vi "LiftControlLoop.vi"() -> ()   [LabVIEW 2014, in "LiftLib.lvlib"]
uses:
  LiftLib.lvlib
  LiftRefs.ctl
  <vilib>/Rock Robotics/WPI/Solenoid/WPI_SolenoidValue.ctl
  <vilib>/addons/control/pid/pid.llb/PID (DBL).vi
  <vilib>/Rock Robotics/Network Tables/SD Write Number.vi
  <vilib>/Rock Robotics/Network Tables/SD Read Boolean.vi
  <vilib>/Rock Robotics/Network Tables/SD Write Boolean.vi
  <vilib>/addons/control/pid/NI_PID_pid.lvlib
  IntakeLib/IntakeLib.lvlib
panel:
  out "LiftRateLast":dbl format="%#_13g"
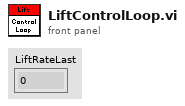
[diagram p1: front panel]
types:
  T1 = typedef "LiftLib.lvlib/LiftRefs.ctl" = enum16{"LiftCim1", "LiftCim2", "LiftEncoder", "LiftLimitSwitch1", "LiftLimitSwitch2"}
  T2 = typedef "WPI_MotorControlDeviceRef.ctl" = cluster{"DeviceStatus":errorcluster, "Type":T3, "PWM":cluster{"Controller":T4, "PWM Channel":T5, "DeadBand":T6}, "CAN":cluster{"Device Number":u8, "Control Mode":T7, "Semaphore":T8, "Max Vout":dbl, "TalonSRX Control Mode":T9}, "Invert":bool, "TransformRef":T10, "InvTransformRef":T10}
  T3 = typedef "WPI_MotorControlType.ctl" = enum16{"PWM", "CAN", "CANTalonSRX"}
  T4 = typedef "FPGA_TypedefDigitalModule.ctl" = enum16{"Controller 1"}
  T5 = typedef "FPGA_DIOPWMChannel.ctl" = enum8{"PWM 0", "PWM 1", "PWM 2", "PWM 3", "PWM 4", "PWM 5", "PWM 6", "PWM 7", "PWM 8", "PWM 9", "PWM MXP 0", "PWM MXP 1", "PWM MXP 2", "PWM MXP 3", "PWM MXP 4", "PWM MXP 5", "PWM MXP 6", "PWM MXP 7", "PWM MXP 8", "PWM MXP 9", "Invalid"}
  T6 = typedef "WPI_PWMDeadband.ctl" = cluster{"Name":string, "maxPositivePwm":i32, "minPositivePwm":i32, "centerPwm":i32, "maxNegativePwm":i32, "minNegativePwm":i32, "angularRange":u16}
  T7 = typedef "WPI_CANJaguar_ControlMode.ctl" = enum8{"Percent VBus", "Current", "Speed", "Position", "Voltage"}
  T8 = typedef "Semaphore RefNum" = refnum<k1>
  T9 = typedef "WPI_CANTalonSRX_APIControlMode.ctl" = enum8{"Percent VBus", "Speed", "Position", "Slave", "Unchanged / Invalid"}
  T10 = typedef "WPI_PWMTransform_ConPane.ctl" = refnum<vi>
  T11 = typedef "WPI_EncoderDevRef.ctl" = cluster{"DevStatus":errorcluster, "EncoderIndex":T12, "CounterIndex":T13, "DistancePerCount":dbl, "Decoding Type":T14}
  T12 = typedef "FPGA_EncoderIdx.ctl" = enum8{"Enc 0", "Enc 1", "Enc 2", "Enc 3", "Enc 4", "Enc 5", "Enc 6", "Enc 7", "Invalid"}
  T13 = typedef "FPGA_CounterCtrSystemIndex.ctl" = enum8{"Ctr 0", "Ctr 1", "Ctr 2", "Ctr 3", "Ctr 4", "Ctr 5", "Ctr 6", "Ctr 7", "Invalid"}
  T14 = typedef "WPI_EncoderType.ctl" = enum16{"1x", "2x", "4x"}
  T15 = typedef "WPI_DigitalInputDevRef.ctl" = cluster{"DevStatus":errorcluster, "DIO Channel":T16, "Controller":T4}
  T16 = typedef "FPGA_DIOChannel.ctl" = enum8{"DIO 0", "DIO 1", "DIO 2", "DIO 3", "DIO 4", "DIO 5", "DIO 6", "DIO 7", "DIO 8", "DIO 9", "DIO MXP 0", "DIO MXP 1", "DIO MXP 2", "DIO MXP 3", "DIO MXP 4", "DIO MXP 5", "DIO MXP 6", "DIO MXP 7", "DIO MXP 8", "DIO MXP 9", "DIO MXP 10", "DIO MXP 11", "DIO MXP 12", "DIO MXP 13", "DIO MXP 14", "DIO MXP 15", "Invalid"}
  T17 = typedef "WPI_SolenoidValue.ctl" = enum16{"Off", "On", "Forward", "Reverse"}
  T18 = cluster{"proportional gain (Kc)":dbl, "integral time (Ti, min)":dbl, "derivative time (Td, min)":dbl}
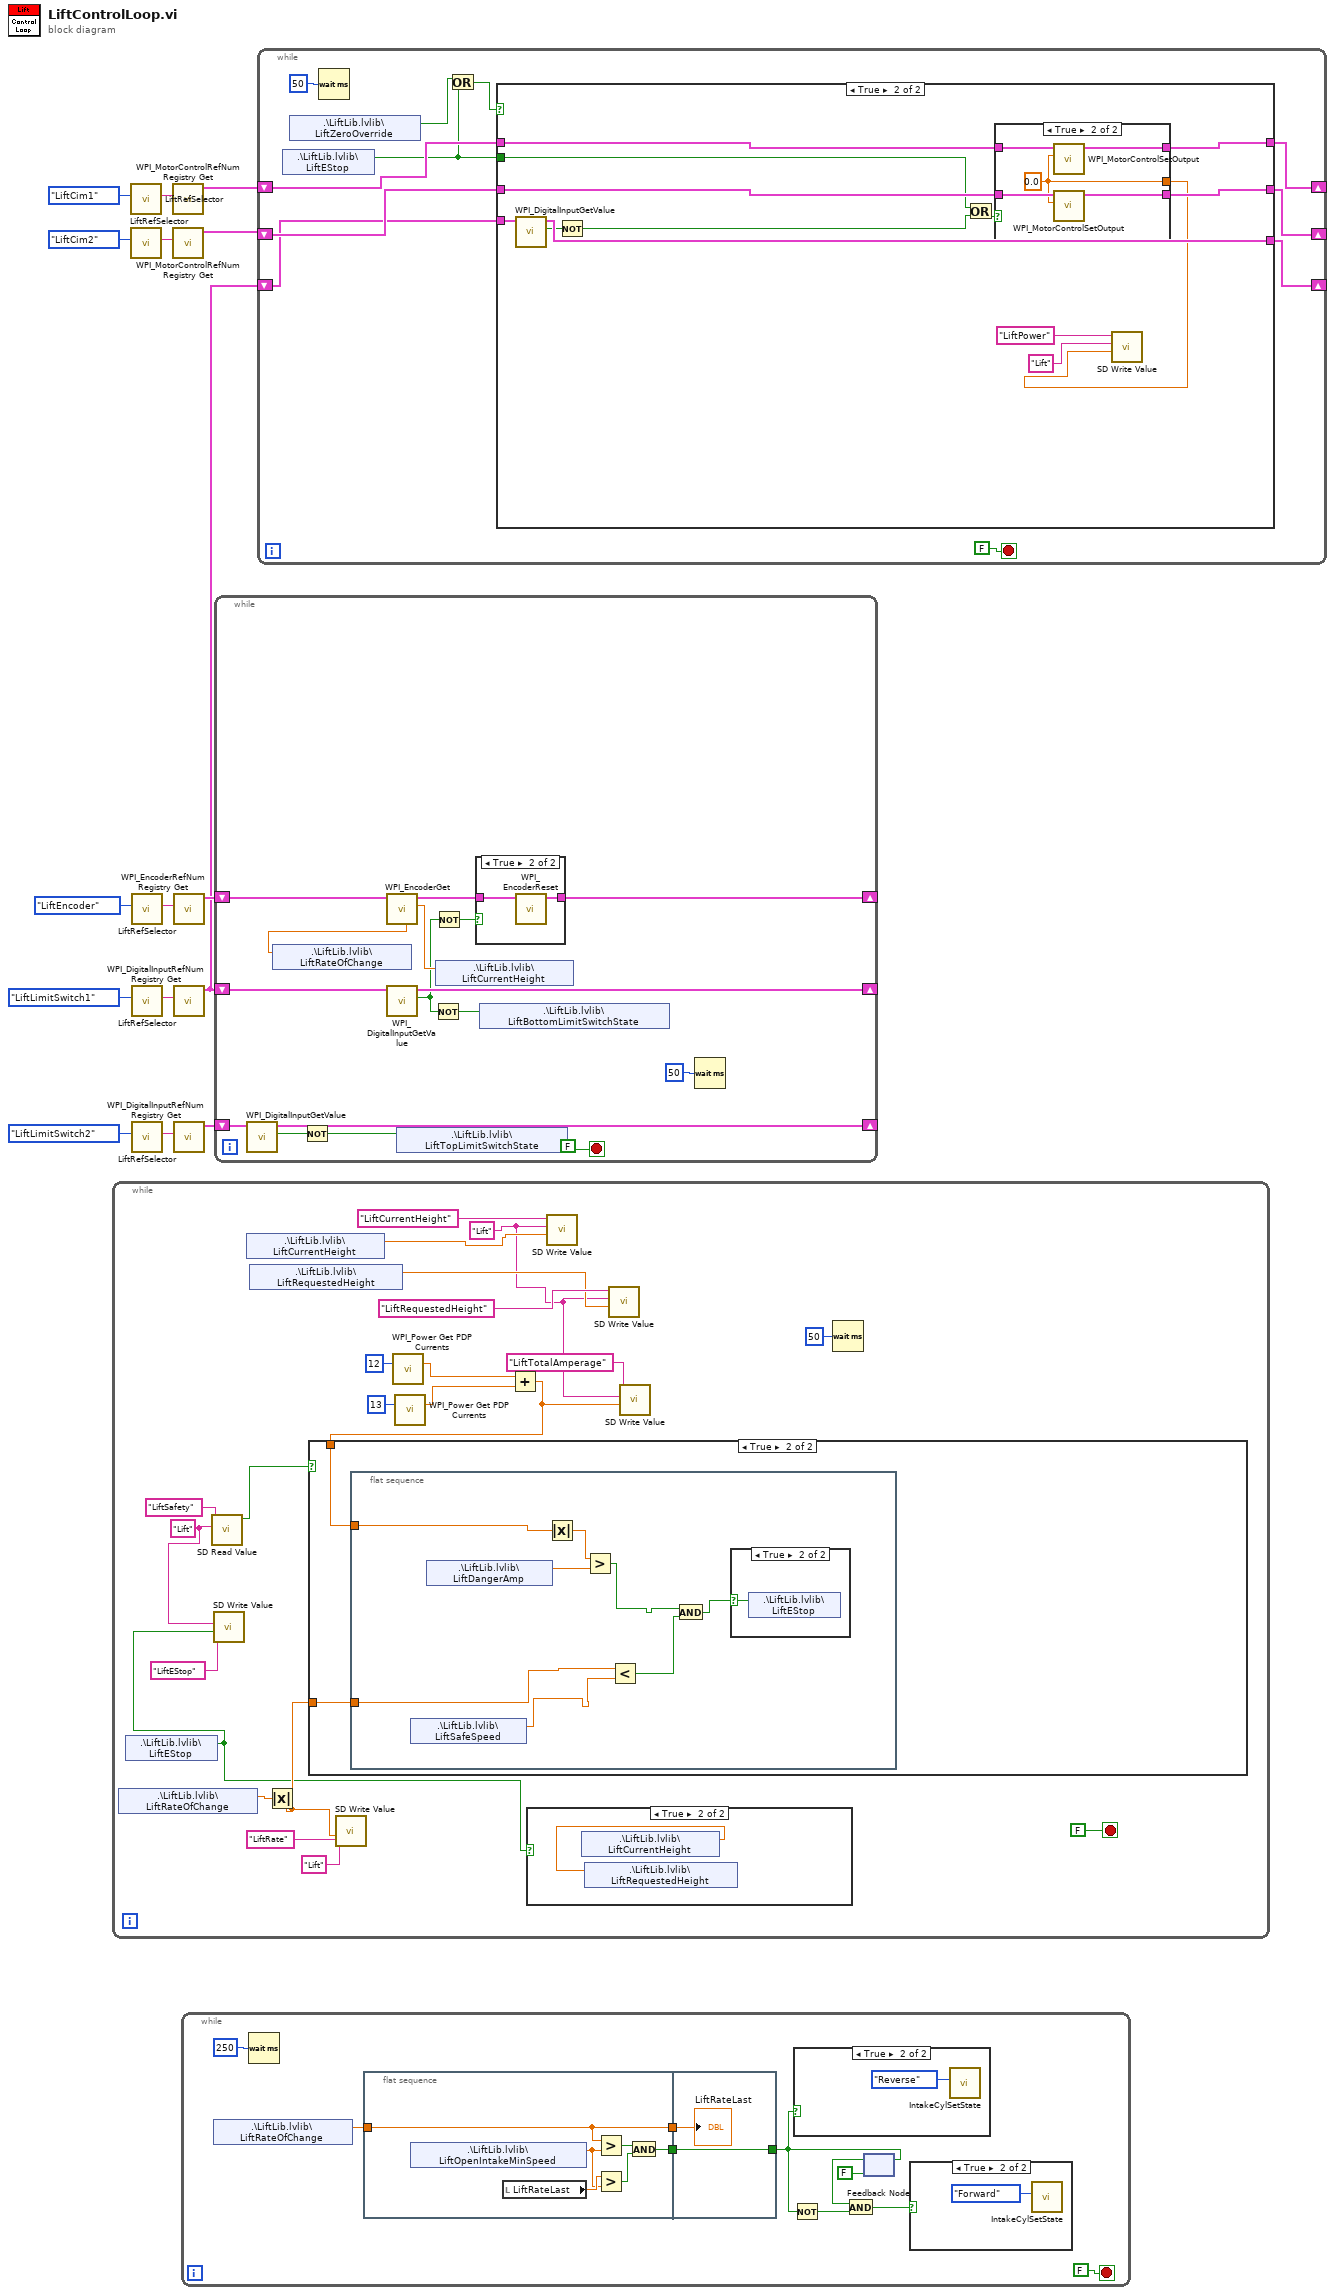
[diagram p0: block diagram]
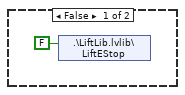
[diagram p5: hidden frame]
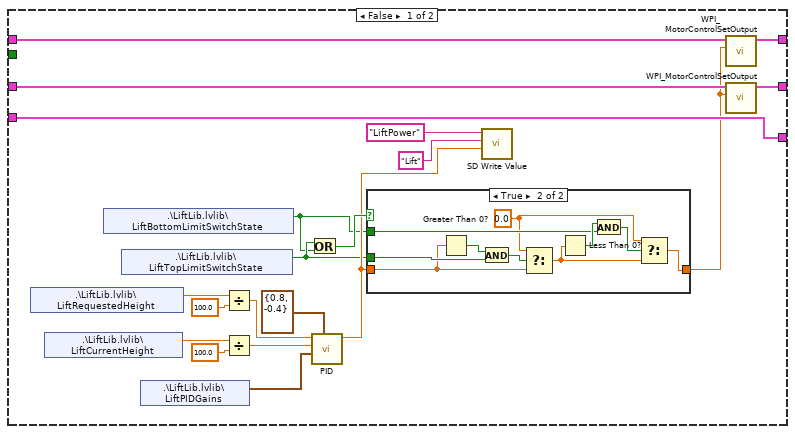
[diagram p8: hidden frame]
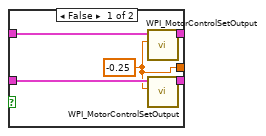
[diagram p10: hidden frame]
diagram:
  n1 = while {
    stop <- FALSE stop-if-true
    w22 = "Lift" ("Table Prefix")
    w27 = "Lift" ("Table Prefix")
    n2 = shared-variable ".\\LiftLib.lvlib\\LiftRateOfChange"() -> (w18:dbl)  [unwired: 1 in, 1 out]
    n3 = shared-variable ".\\LiftLib.lvlib\\LiftEStop"() -> (w16:bool)  [unwired: 1 in, 1 out]
    n4 = call-poly <vilib>:"SD Read Value.vi"("Table Prefix"=w22, "Name"="LiftSafety") -> ("Boolean"=w23:bool)  [unwired: 7 in, 2 out]
    n5 = call-poly <vilib>:"SD Write Value.vi"("Boolean"=w16, "Table Prefix"=w22, "Name"="LiftEStop") -> ()  [unwired: 7 in, 2 out]
    n6 = shared-variable ".\\LiftLib.lvlib\\LiftCurrentHeight"() -> (w34:dbl)  [unwired: 1 in, 1 out]
    n7 = shared-variable ".\\LiftLib.lvlib\\LiftRequestedHeight"() -> (w35:dbl)  [unwired: 1 in, 1 out]
    n8 = Absolute Value(x=w18) -> (abs(x)=w17:dbl)
    n9 = call-poly <vilib>:"SD Write Value.vi"("Numeric"=w17, "Table Prefix"="Lift", "Name"="LiftRate") -> ()  [unwired: 7 in, 2 out]
    n10 = call <vilib>:"WPI_Power Get PDP Currents.vi"("PDP Channel"=12) -> ("current (A)"=w29:dbl)  [unwired: 12 in, 2 out]
    n11 = call <vilib>:"WPI_Power Get PDP Currents.vi"("PDP Channel"=13) -> ("current (A)"=w28:dbl)  [unwired: 12 in, 2 out]
    n12 = Add(x=w29, y=w28) -> (x+y=w25:dbl)
    n13 = case shown="True" w23 {
      tunnel: w25 -> [_ w41]
      tunnel: w17 -> [_ w40]
      frame False {
        n14 = shared-variable ".\\LiftLib.lvlib\\LiftEStop"(FALSE ("LiftEStop")) -> ()  [unwired: 1 in, 1 out]
      }
      frame True {
        n15 = flat-sequence {
          tunnel: w41 -> [w42]
          tunnel: w40 -> [w44]
          frame #0 {
            n16 = shared-variable ".\\LiftLib.lvlib\\LiftSafeSpeed"() -> (w45:dbl)  [unwired: 1 in, 1 out]
            n17 = shared-variable ".\\LiftLib.lvlib\\LiftDangerAmp"() -> (w48:dbl)  [unwired: 1 in, 1 out]
            n18 = Absolute Value(x=w42) -> (abs(x)=w49:dbl)
            n19 = Greater?(x=w49, y=w48) -> (0:w43:bool)
            n20 = Less?(x=w44, y=w45) -> (x < y?=w46:bool)
            n21 = And(x=w43, y=w46) -> (x .and. y?=w47:bool)
            n22 = case shown="True" w47 {
              selector: w47 -> [_ w50]
              frame False {
              }
              frame True {
                n23 = shared-variable ".\\LiftLib.lvlib\\LiftEStop"(w50) -> ()  [unwired: 1 in, 1 out]
              }
            }
          }
        }
      }
    }
    n24 = case shown="True" w16 {
      frame False {
      }
      frame True {
        n25 = shared-variable ".\\LiftLib.lvlib\\LiftCurrentHeight"() -> (w38:dbl)  [unwired: 1 in, 1 out]
        n26 = shared-variable ".\\LiftLib.lvlib\\LiftRequestedHeight"(w38) -> ()  [unwired: 1 in, 1 out]
      }
    }
    n27 = call-poly <vilib>:"SD Write Value.vi"("Numeric"=w34, "Table Prefix"=w27, "Name"="LiftCurrentHeight") -> ()  [unwired: 7 in, 2 out]
    n28 = call-poly <vilib>:"SD Write Value.vi"("Numeric"=w35, "Table Prefix"=w27, "Name"="LiftRequestedHeight") -> ()  [unwired: 7 in, 2 out]
    n29 = call-poly <vilib>:"SD Write Value.vi"("Numeric"=w25, "Table Prefix"=w27, "Name"="LiftTotalAmperage") -> ()  [unwired: 7 in, 2 out]
    n30 = Wait (ms)(milliseconds to wait=u32 50) -> ()  [unwired: 1 out]
  }
  n31 = call "LiftRefSelector.vi"("LiftRefs"=LiftRefs."LiftCim1") -> ("String"=w5:string)  [unwired: 10 in]
  n32 = call "LiftRefSelector.vi"("LiftRefs"=LiftRefs."LiftCim2") -> ("String"=w4:string)  [unwired: 10 in]
  n33 = call "LiftRefSelector.vi"("LiftRefs"=LiftRefs."LiftEncoder") -> ("String"=w10:string)  [unwired: 10 in]
  n34 = call "LiftRefSelector.vi"("LiftRefs"=LiftRefs."LiftLimitSwitch1") -> ("String"=w15:string)  [unwired: 10 in]
  n35 = call "LiftRefSelector.vi"("LiftRefs"=LiftRefs."LiftLimitSwitch2") -> ("String"=w14:string)  [unwired: 10 in]
  n36 = call <vilib>:"WPI_MotorControlRefNum Registry Get.vi"("refnum name"=w5) -> ("MotorControlDevRef"=w3:T2)  [unwired: 9 in, 1 out]
  n37 = call <vilib>:"WPI_MotorControlRefNum Registry Get.vi"("refnum name"=w4) -> ("MotorControlDevRef"=w2:T2)  [unwired: 9 in, 1 out]
  n38 = call <vilib>:"WPI_EncoderRefNum Registry Get.vi"("refnum name"=w10) -> ("EncoderDevRef"=w9:T11)  [unwired: 9 in, 1 out]
  n39 = call <vilib>:"WPI_DigitalInputRefNum Registry Get.vi"("refnum name"=w15) -> ("DigitalInputDevRef"=w1:T15)  [unwired: 9 in, 1 out]
  n40 = call <vilib>:"WPI_DigitalInputRefNum Registry Get.vi"("refnum name"=w14) -> ("DigitalInputDevRef"=w8:T15)  [unwired: 9 in, 1 out]
  n41 = while {
    stop <- FALSE stop-if-true
    n42 = shared-variable ".\\LiftLib.lvlib\\LiftRateOfChange"() -> (w51:dbl)  [unwired: 1 in, 1 out]
    n43 = Wait (ms)(milliseconds to wait=u32 250) -> ()  [unwired: 1 out]
    n44 = flat-sequence {
      tunnel: w51 -> [w62]
      tunnel: [w61] -> w60
      tunnel: [w62] -> w59
      tunnel: [w68] -> w57
      tunnel: w60 -> [w68]
      tunnel: w59 -> [w67]
      frame #0 {
        n45 = shared-variable ".\\LiftLib.lvlib\\LiftOpenIntakeMinSpeed"() -> (w65:dbl)  [unwired: 1 in, 1 out]
        n46 = local read "LiftRateLast"() -> (w66:dbl)
        n47 = Greater?(x=w62, y=w65) -> (0:w64:bool)
        n48 = Greater?(x=w66, y=w65) -> (0:w63:bool)
        n49 = And(x=w64, y=w63) -> (x .and. y?=w61:bool)
      }
      frame #1 {
        "LiftRateLast" <- w67
      }
    }
    n50 = Not(x=w57) -> (.not. x?=w56:bool)
    n51 = case shown="True" w57 {
      frame False {
      }
      frame True {
        n52 = call "IntakeCylSetState.vi"("IntakeCylState"=WPI_SolenoidValue."Reverse") -> ()  [unwired: 11 in]
      }
    }
    n53 = feedback #1(FALSE) -> (w55:bool)
    n54 = And(x=w55, y=w56) -> (x .and. y?=w54:bool)
    n55 = feedback-in #1(w57) -> ()
    n56 = case shown="True" w54 {
      frame False {
      }
      frame True {
        n57 = call "IntakeCylSetState.vi"("IntakeCylState"=WPI_SolenoidValue."Forward") -> ()  [unwired: 11 in]
      }
    }
  }
  n58 = while {
    shift-right: [w81] -> _
    shift-left: w1 -> [w85]
    shift-right: [w80] -> _
    shift-left: w8 -> [w86]
    shift-right: [w84] -> _
    shift-left: w9 -> [w83]
    stop <- FALSE stop-if-true
    n59 = call <vilib>:"WPI_DigitalInputGetValue.vi"("DigitalInputDevRef"=w86) -> ("Value"=w74:bool, "DigitalInputDevRef"=w80:T15)  [unwired: 8 in, 1 out]
    n60 = Not(x=w74) -> (.not. x?=w73:bool)
    n61 = call <vilib>:"WPI_EncoderGet.vi"("EncoderDevRef"=w83) -> ("Distance"=w76:dbl, "EncoderDevRef"=w82:T11, "Rate"=w71:dbl)  [unwired: 5 in, 3 out]
    n62 = shared-variable ".\\LiftLib.lvlib\\LiftRateOfChange"(w71) -> ()  [unwired: 1 in, 1 out]
    n63 = call <vilib>:"WPI_DigitalInputGetValue.vi"("DigitalInputDevRef"=w85) -> ("Value"=w75:bool, "DigitalInputDevRef"=w81:T15)  [unwired: 8 in, 1 out]
    n64 = shared-variable ".\\LiftLib.lvlib\\LiftTopLimitSwitchState"(w73) -> ()  [unwired: 1 in, 1 out]
    n65 = Not(x=w75) -> (.not. x?=w72:bool)
    n66 = Not(x=w75) -> (.not. x?=w77:bool)
    n67 = shared-variable ".\\LiftLib.lvlib\\LiftCurrentHeight"(w76) -> ()  [unwired: 1 in, 1 out]
    n68 = case shown="True" w77 {
      tunnel: w82 -> [w87 w89]
      tunnel: [w87 w88] -> w84
      frame False {
      }
      frame True {
        n69 = call <vilib>:"WPI_EncoderReset.vi"("EncoderDevRef"=w89) -> ("EncoderDevRef"=w88:T11)  [unwired: 9 in, 1 out]
      }
    }
    n70 = shared-variable ".\\LiftLib.lvlib\\LiftBottomLimitSwitchState"(w72) -> ()  [unwired: 1 in, 1 out]
    n71 = Wait (ms)(milliseconds to wait=u32 50) -> ()  [unwired: 1 out]
  }
  n72 = while {
    shift-right: [w98] -> _
    shift-left: w3 -> [w96]
    shift-right: [w97] -> _
    shift-left: w2 -> [w95]
    shift-right: [w93] -> _
    shift-left: w1 -> [w94]
    stop <- FALSE stop-if-true
    n73 = shared-variable ".\\LiftLib.lvlib\\LiftEStop"() -> (w90:bool)  [unwired: 1 in, 1 out]
    n74 = shared-variable ".\\LiftLib.lvlib\\LiftZeroOverride"() -> (w92:bool)  [unwired: 1 in, 1 out]
    n75 = Wait (ms)(milliseconds to wait=u32 50) -> ()  [unwired: 1 out]
    n76 = Or(x=w92, y=w90) -> (x .or. y?=w91:bool)
    n77 = case shown="True" w91 {
      tunnel: [w118 w140] -> w98
      tunnel: [w117 w138] -> w97
      tunnel: w96 -> [w116 w141]
      tunnel: w95 -> [w105 w139]
      tunnel: w94 -> [w107 w144]
      tunnel: [w107 w143] -> w93
      tunnel: w90 -> [_ w135]
      frame False {
        n78 = shared-variable ".\\LiftLib.lvlib\\LiftRequestedHeight"() -> (w115:dbl)  [unwired: 1 in, 1 out]
        n79 = shared-variable ".\\LiftLib.lvlib\\LiftCurrentHeight"() -> (w111:dbl)  [unwired: 1 in, 1 out]
        n80 = shared-variable ".\\LiftLib.lvlib\\LiftBottomLimitSwitchState"() -> (w101:bool)  [unwired: 1 in, 1 out]
        n81 = shared-variable ".\\LiftLib.lvlib\\LiftTopLimitSwitchState"() -> (w102:bool)  [unwired: 1 in, 1 out]
        n82 = shared-variable ".\\LiftLib.lvlib\\LiftPIDGains"() -> (w119:T18)  [unwired: 1 in, 1 out]
        n83 = Divide(x=w115, y=100.0) -> (x/y=w113:dbl)
        n84 = Divide(x=w111, y=100.0) -> (x/y=w110:dbl)
        n85 = Or(x=w102, y=w101) -> (x .or. y?=w106:bool)
        n86 = call-poly <vilib>:"PID.vi"("output range"=cluster{"output high":dbl, "output low":dbl} {"output high"=0.8, "output low"=-0.4}, "PID gains"=w119, "process variable"=w110, "setpoint"=w113) -> ("output"=w104:dbl)  [unwired: 6 in, 1 out]
        n87 = case shown="True" w106 {
          tunnel: w104 -> [w121 w128]
          tunnel: [w121 w122] -> w103
          tunnel: w102 -> [_ w130]
          tunnel: w101 -> [_ w126]
          frame False {
          }
          frame True {
            w124 = 0.0 ("t")
            n88 = Greater Than 0?(x=w128) -> (x > 0?=w131:bool)
            n89 = And(x=w131, y=w130) -> (x .and. y?=w129:bool)
            n90 = Select(t=w124, s=w129, f=w128) -> (s? t:f=w123:dbl)
            n91 = Less Than 0?(x=w123) -> (x < 0?=w127:bool)
            n92 = And(x=w127, y=w126) -> (x .and. y?=w125:bool)
            n93 = Select(t=w124, s=w125, f=w123) -> (s? t:f=w122:dbl)
          }
        }
        n94 = call-poly <vilib>:"SD Write Value.vi"("Numeric"=w104, "Table Prefix"="Lift", "Name"="LiftPower") -> ()  [unwired: 7 in, 2 out]
        n95 = call <vilib>:"WPI_MotorControlSetOutput.vi"("Output"=w103, "MotorControlDevRef"=w116) -> ("MotorControlDevRef"=w118:T2)  [unwired: 7 in, 2 out]
        n96 = call <vilib>:"WPI_MotorControlSetOutput.vi"("Output"=w103, "MotorControlDevRef"=w105) -> ("MotorControlDevRef"=w117:T2)  [unwired: 7 in, 2 out]
      }
      frame True {
        n97 = call <vilib>:"WPI_DigitalInputGetValue.vi"("DigitalInputDevRef"=w144) -> ("Value"=w142:bool, "DigitalInputDevRef"=w143:T15)  [unwired: 8 in, 1 out]
        n98 = Not(x=w142) -> (.not. x?=w136:bool)
        n99 = Or(x=w135, y=w136) -> (x .or. y?=w137:bool)
        n100 = case shown="True" w137 {
          tunnel: w141 -> [w149 w154]
          tunnel: [w148 w153] -> w140
          tunnel: w139 -> [w147 w151]
          tunnel: [w146 w152] -> w138
          tunnel: [w145 w150] -> w132
          frame False {
            w145 = -0.25 ("Output")
            n101 = call <vilib>:"WPI_MotorControlSetOutput.vi"("Output"=w145, "MotorControlDevRef"=w149) -> ("MotorControlDevRef"=w148:T2)  [unwired: 7 in, 2 out]
            n102 = call <vilib>:"WPI_MotorControlSetOutput.vi"("Output"=w145, "MotorControlDevRef"=w147) -> ("MotorControlDevRef"=w146:T2)  [unwired: 7 in, 2 out]
          }
          frame True {
            w150 = 0.0 ("Output")
            n103 = call <vilib>:"WPI_MotorControlSetOutput.vi"("Output"=w150, "MotorControlDevRef"=w154) -> ("MotorControlDevRef"=w153:T2)  [unwired: 7 in, 2 out]
            n104 = call <vilib>:"WPI_MotorControlSetOutput.vi"("Output"=w150, "MotorControlDevRef"=w151) -> ("MotorControlDevRef"=w152:T2)  [unwired: 7 in, 2 out]
          }
        }
        n105 = call-poly <vilib>:"SD Write Value.vi"("Numeric"=w132, "Table Prefix"="Lift", "Name"="LiftPower") -> ()  [unwired: 7 in, 2 out]
      }
    }
  }
